vi "Connection Count FGV.vi"(8 "error in (no error)":errorcluster, 11 "Action (Read)":enum16{"Read", "Inc", "Dec"}(ring)) -> (0 "error out":errorcluster, 2 "Count":u32)   [LabVIEW 2017]
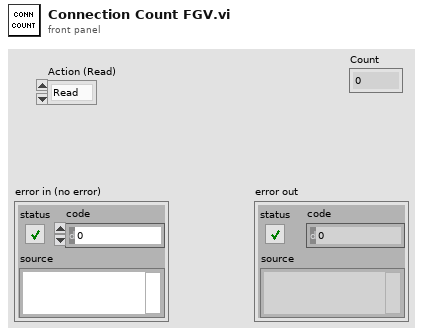
[diagram p1: front panel]
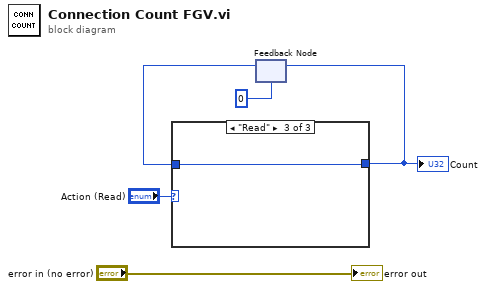
[diagram p0: block diagram]
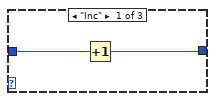
[diagram p2: hidden frame]
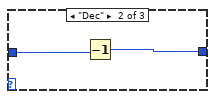
[diagram p3: hidden frame]
diagram:
  n1 = feedback #1(u32 0) -> (w3:u32)
  n2 = case shown="\"Read\"" "Action (Read)" {
    tunnel: [w7 w9 w10] -> w4
    tunnel: w3 -> [w6 w8 w10]
    frame "Inc" {
      n3 = Increment(x=w6) -> (x+1=w7:u32)
    }
    frame "Dec" {
      n4 = Decrement(x=w8) -> (x-1=w9:u32)
    }
    frame "Read" {
    }
  }
  "Count" <- w4
  n5 = feedback-in #1(w4) -> ()
  "error out" <- "error in (no error)"
